vi "config_Peak.vi"(6 "tipo_ciclo":string, 8 "error in (no error)":errorcluster, 10 "Amplitud (Vrms)":dbl, 11 "Frec (Hz)":dbl) -> (0 "error out":errorcluster, 3 "DS360 out":refnum<class "DS360.lvclass">)   [LabVIEW 2019, in "DS360.lvclass"]
uses:
  DS360.lvclass
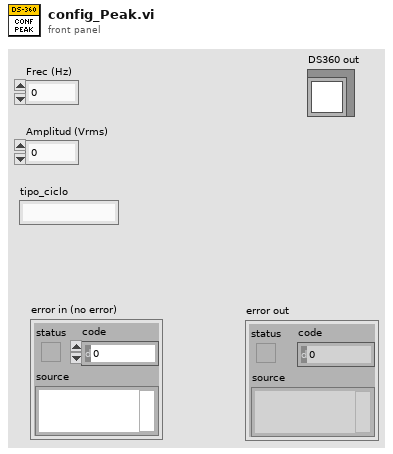
[diagram p1: front panel]
types:
  T1 = cluster{"error":bool, "code":i32, "source":string}
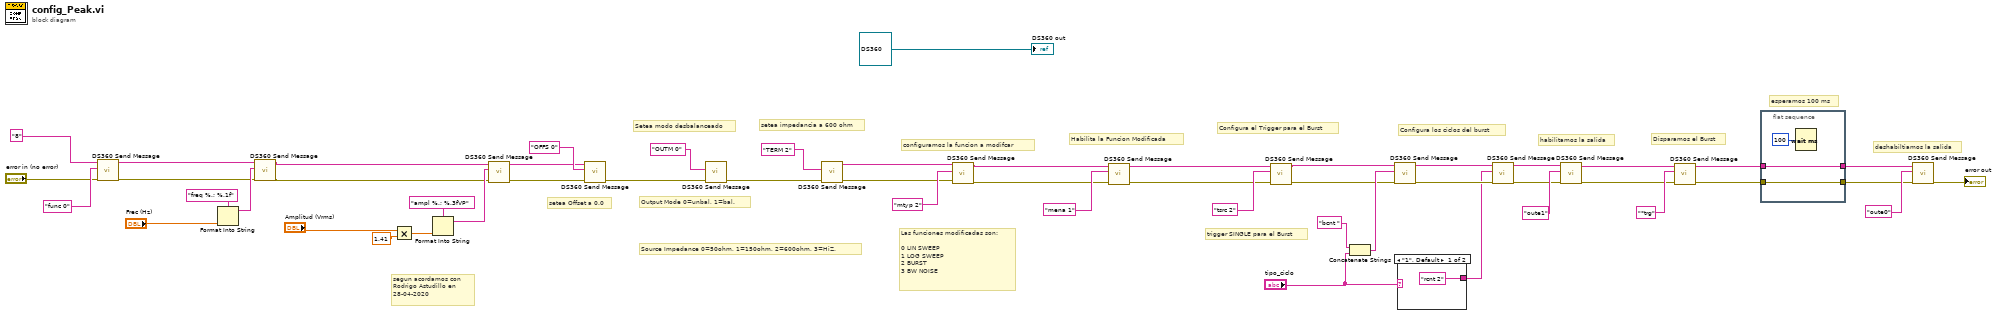
[diagram p0: block diagram]
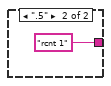
[diagram p2: hidden frame]
diagram:
  # "Las funciones modificadas son:\n\n0 LIN SWEEP\n1 LOG SWEEP\n2 BURST\n3 BW NOISE"
  # "configuramos la funcion a modifcar"
  # "Source Impedance 0=50ohm, 1=150ohm, 2=600ohm, 3=HiZ."
  # "Output Mode 0=unbal, 1=bal."
  # "setea impedancia a 600 ohm"
  # "Setea modo desbalanceado"
  # "setea Offset a 0.0"
  # "deshabiltiamos la salida"
  # "esperamos 100 ms"
  # "habilitamos la salida"
  # "Disparamos el Burst"
  # "Configura los ciclos del burst"
  # "trigger SINGLE para el Burst"
  # "Configura el Trigger para el Burst"
  # "Habilita la Funcion Modificada"
  # "segun acordamos con\nRodrigo Astudillo en\n28-04-2020"
  n1 = call <instrlib>:"DS360 Send Message.vi"("address string"="8" ("write buffer"), "write buffer"="func 0", "error in"="error in (no error)") -> ("address out"=w28:string, "error out"=w27:T1)  [unwired: 3 in, 2 out]
  n2 = Format Into String(format string="freq %.; %.1f" ("write buffer"), "Frec (Hz)") -> (resulting string=w50:string)  [unwired: 2 in, 1 out]
  n3 = call <instrlib>:"DS360 Send Message.vi"("address string"=w28, "write buffer"=w50, "error in"=w27) -> ("address out"=w26:string, "error out"=w25:T1)  [unwired: 3 in, 2 out]
  n4 = Multiply(x="Amplitud (Vrms)", y=1.41) -> (x*y=w48:dbl)
  n5 = Format Into String(format string="ampl %.; %.3fVP" ("write buffer"), w48) -> (resulting string=w46:string)  [unwired: 2 in, 1 out]
  n6 = call <instrlib>:"DS360 Send Message.vi"("address string"=w26, "write buffer"=w46, "error in"=w25) -> ("address out"=w4:string, "error out"=w3:T1)  [unwired: 3 in, 2 out]
  n7 = call <instrlib>:"DS360 Send Message.vi"("address string"=w4, "write buffer"="OFFS 0", "error in"=w3) -> ("error out"=w8:T1)  [unwired: 3 in, 3 out]
  n8 = call <instrlib>:"DS360 Send Message.vi"("write buffer"="OUTM 0", "error in"=w8) -> ("error out"=w7:T1)  [unwired: 4 in, 3 out]
  n9 = call <instrlib>:"DS360 Send Message.vi"("write buffer"="TERM 2", "error in"=w7) -> ("address out"=w2:string, "error out"=w1:T1)  [unwired: 4 in, 2 out]
  n10 = call <instrlib>:"DS360 Send Message.vi"("address string"=w2, "write buffer"="mtyp 2", "error in"=w1) -> ("address out"=w24:string, "error out"=w23:T1)  [unwired: 3 in, 2 out]
  n11 = call <instrlib>:"DS360 Send Message.vi"("address string"=w24, "write buffer"="mena 1", "error in"=w23) -> ("address out"=w22:string, "error out"=w21:T1)  [unwired: 3 in, 2 out]
  n12 = call <instrlib>:"DS360 Send Message.vi"("address string"=w22, "write buffer"="tsrc 2", "error in"=w21) -> ("address out"=w20:string, "error out"=w19:T1)  [unwired: 3 in, 2 out]
  n13 = Concatenate Strings("bcnt " ("write buffer"), "tipo_ciclo") -> (w38:string)
  n14 = call <instrlib>:"DS360 Send Message.vi"("address string"=w20, "write buffer"=w38, "error in"=w19) -> ("address out"=w40:string, "error out"=w41:T1)  [unwired: 3 in, 2 out]
  n15 = case shown="\"1\", Default" "tipo_ciclo" {
    tunnel: ["rcnt 2" ("write buffer") "rcnt 1" ("write buffer")] -> w39
    frame "1", Default {
    }
    frame ".5" {
    }
  }
  n16 = call <instrlib>:"DS360 Send Message.vi"("address string"=w40, "write buffer"=w39, "error in"=w41) -> ("address out"=w18:string, "error out"=w17:T1)  [unwired: 3 in, 2 out]
  n17 = call <instrlib>:"DS360 Send Message.vi"("address string"=w18, "write buffer"="oute1", "error in"=w17) -> ("address out"=w16:string, "error out"=w15:T1)  [unwired: 3 in, 2 out]
  n18 = call <instrlib>:"DS360 Send Message.vi"("address string"=w16, "write buffer"="*trg", "error in"=w15) -> ("address out"=w13:string, "error out"=w14:T1)  [unwired: 3 in, 2 out]
  n19 = flat-sequence {
    tunnel: w14 -> [w56]
    tunnel: w13 -> [w55]
    tunnel: [w56] -> w11
    tunnel: [w55] -> w12
    frame #0 {
      n20 = Wait (ms)(milliseconds to wait=u32 100) -> ()  [unwired: 1 out]
    }
  }
  n21 = call <instrlib>:"DS360 Send Message.vi"("address string"=w12, "write buffer"="oute0", "error in"=w11) -> ("error out"=→"error out":T1)  [unwired: 3 in, 3 out]
  "DS360 out" <- refnum<class "DS360.lvclass"> refnum ("DS360 in")
